vi "Close.vi"(8 "error in (no error)":errorcluster, 11 "SQLite Database in":refnum<class "SQLite Database.lvclass">) -> (0 "error out":errorcluster, 3 "SQLite Database out":refnum<class "SQLite Database.lvclass">)   [LabVIEW 2019, in "TSC Event Logger (SQL).lvlib" / "SQLite Database.lvclass"]
uses:
  SQLite Database.lvclass
  SQLite Database.lvclass/SQLite Database.ctl
  <vilib>/drjdpowell/SQLite Library/SQL Statement/SQL Statement.lvclass/SQL Statement.ctl
  <vilib>/drjdpowell/SQLite Library/SQL Connection/Connection.lvclass
  <vilib>/drjdpowell/SQLite Library/SQL Statement/SQL Statement.lvclass
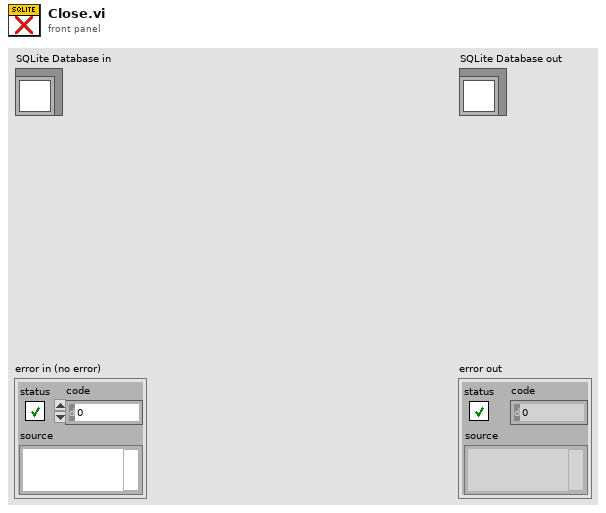
[diagram p1: front panel]
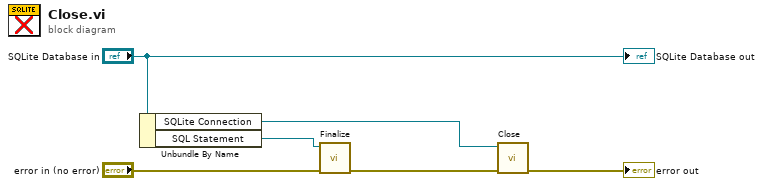
[diagram p0: block diagram]
diagram:
  n1 = Unbundle By Name("SQLite Database in") -> ("SQLite Connection"=w3:refnum<class "Connection.lvclass">, "SQL Statement"=w1:refnum<class "SQL Statement.lvclass">)
  n2 = call <vilib>:"Finalize.vi"("error in (no error)"="error in (no error)", "SQL Statement in"=w1) -> ("error out"=w2:errorcluster)  [unwired: 9 in]
  n3 = call-dynamic "Close.vi"("error in (no error)"=w2, "SQLite Connection in"=w3) -> ("error out"=→"error out":errorcluster)  [unwired: 9 in]
  "SQLite Database out" <- "SQLite Database in"
